vi "Numerical Offset and Gain.vi"(0 "Signal 1 Offset":dbl[unit] min=-5.0 max=5.0, 1 "Signal 2 Offset":dbl[unit] min=-5.0 max=5.0, 2 "Signal 1 Gain":dbl, 3 "Signal 2 Gain":dbl, 4 "Input Data":dbl[][](array[numeric])) -> (5 "Output Data":dbl[][](array[numeric]))   [LabVIEW 2009]
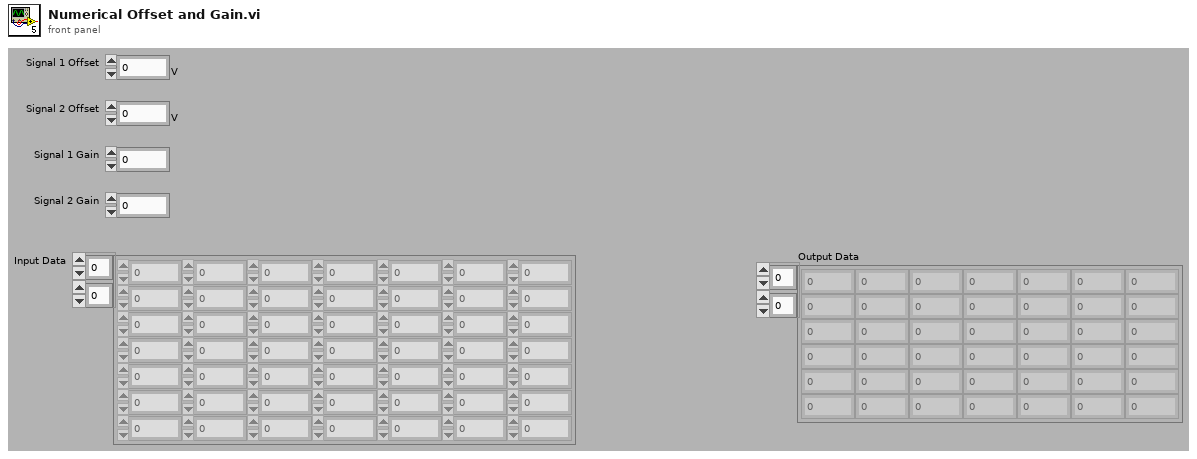
[diagram p1: front panel]
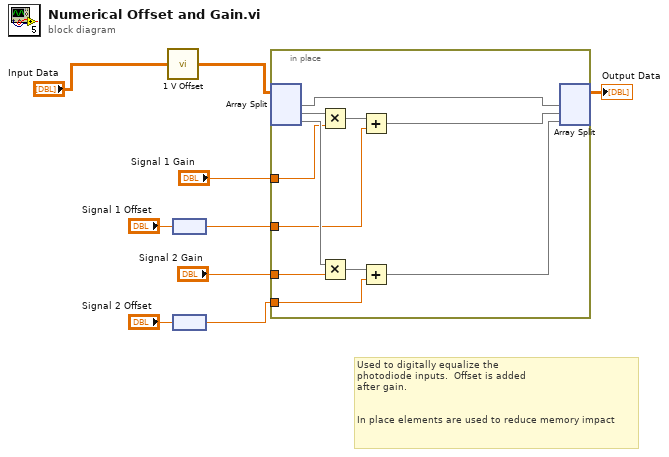
[diagram p0: block diagram]
diagram:
  # "Used to digitally equalize the \nphotodiode inputs.  Offset is added\nafter gain.\n\n\nIn place elements are used to reduce memory impact"
  n1 = call "1 V Offset.vi"("Input Data"="Input Data") -> ("Output Data"=w5:dbl[][])
  n2 = node("Signal 1 Offset") -> (w1:dbl)
  n3 = node("Signal 2 Offset") -> (w4:dbl)
  n4 = in-place {
    in-place-border: w4 -> [w12]
    in-place-border: w1 -> [w13]
    in-place-border: "Signal 1 Gain" -> [w11]
    in-place-border: "Signal 2 Gain" -> [w10]
    n5 = in-place-split #1(w5) -> (w14:dbl[][], w20:dbl[][], w16:dbl[][])  [unwired: 2 in]
    n6 = Multiply(x=w20, y=w11) -> (x*y=w18:dbl[][])
    n7 = Multiply(x=w16, y=w10) -> (x*y=w17:dbl[][])
    n8 = Add(x=w18, y=w13) -> (x+y=w19:dbl[][])
    n9 = Add(x=w17, y=w12) -> (x+y=w15:dbl[][])
    n10 = in-place-split #1(w14, w19, w15) -> (→"Output Data":dbl[][])  [unwired: 2 out]
  }
